vi "zadanie_3.vi"() -> ()   [LabVIEW 2020]
panel:
  out "1":bool
  out "2":bool
  out "4":bool
  out "8":bool
  in  "Numeric":dbl min=0.0 max=15.0
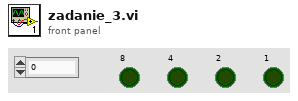
[diagram p1: front panel]
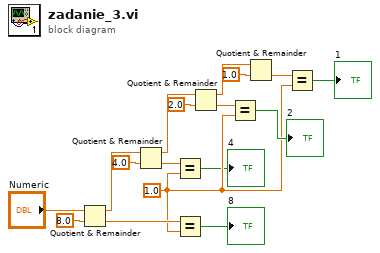
[diagram p0: block diagram]
diagram:
  w3 = 1.0
  n1 = Quotient & Remainder(x="Numeric", y=8.0) -> (x-y*floor(x/y)=w12:dbl, floor(x/y)=w9:dbl)
  n2 = Quotient & Remainder(x=w12, y=4.0) -> (x-y*floor(x/y)=w10:dbl, floor(x/y)=w7:dbl)
  n3 = Equal?(x=w7, y=w3) -> (x = y?=→"4":bool)
  n4 = Equal?(x=w9, y=w3) -> (x = y?=→"8":bool)
  n5 = Quotient & Remainder(x=w10, y=2.0) -> (x-y*floor(x/y)=w11:dbl, floor(x/y)=w6:dbl)
  n6 = Equal?(x=w6, y=w3) -> (x = y?=→"2":bool)
  n7 = Quotient & Remainder(x=w11, y=1.0) -> (floor(x/y)=w4:dbl)  [unwired: 1 out]
  n8 = Equal?(x=w4, y=w3) -> (x = y?=→"1":bool)
